vi "Accelerometer_status.vi"(6 "Number":i32, 10 "Acc_offset":dbl=0.0015, 11 "Accelerometer":sgl[](array[numeric])=array[5000 elements]) -> (2 "Accelerometer_status":string, 3 "Accelerometer":bool)   [LabVIEW 2015]
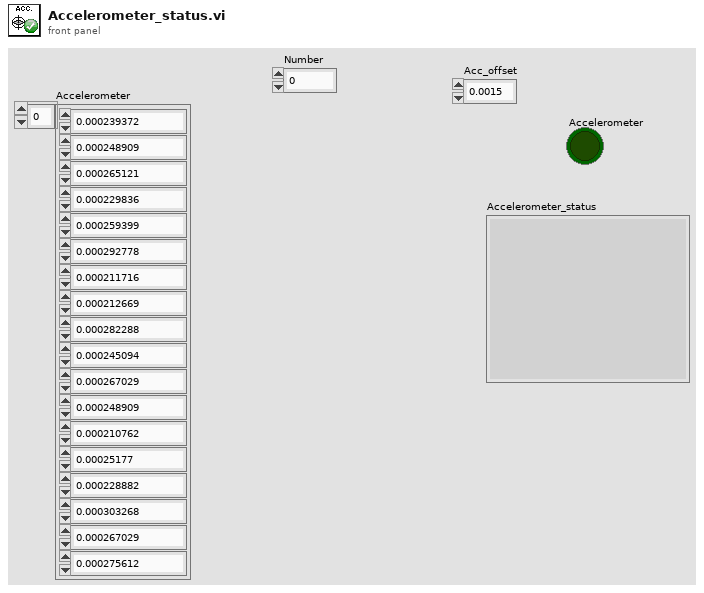
[diagram p1: front panel]
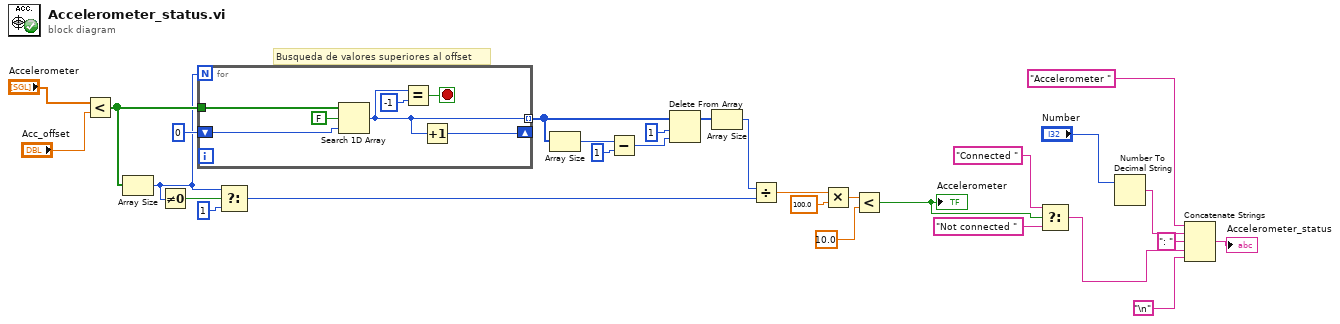
[diagram p0: block diagram]
diagram:
  # "Busqueda de valores superiores al offset"
  n1 = Less?(x="Accelerometer", y="Acc_offset") -> (x < y?=w29:bool[])
  n2 = Array Size(array=w29) -> (size(s)=w21:i32)
  n3 = Not Equal To 0?(x=w21) -> (x != 0?=w26:bool)
  n4 = for {
    N: w21 -> [_]
    tunnel: w29 -> [w36]
    tunnel: [w31] -> w15 mode=indexing
    shift-right: [w30] -> _
    shift-left: 0 ("index of element") -> [w32]
    stop <- w34 stop-if-true
    n5 = Search 1D Array(1D array=w36, element=FALSE, start index (0)=w32) -> (index of element=w31:i32)
    n6 = Equal?(x=w31, y=-1) -> (x = y?=w34:bool)
    n7 = Increment(x=w31) -> (x+1=w30:i32)
  }
  n8 = Select(t=w21, s=w26, f=1) -> (s? t:f=w27:i32)
  n9 = Array Size(array=w15) -> (size(s)=w19:i32)
  n10 = Subtract(x=w19, y=1 ("length")) -> (x-y=w17:i32)
  n11 = Delete From Array(array=w15, length=1, index=w17) -> (array with subset deleted=w14:i32[])  [unwired: 1 out]
  n12 = Array Size(array=w14) -> (size(s)=w22:i32)
  n13 = Divide(x=w22, y=w27) -> (x/y=w24:dbl)
  n14 = Multiply(x=w24, y=100.0) -> (x*y=w20:dbl)
  n15 = Less?(x=w20, y=10.0) -> (x < y?=w13:bool)
  "Accelerometer" <- w13
  n16 = Select(t="Connected " ("string"), s=w13, f="Not connected " ("string")) -> (s? t:f=w10:string)
  n17 = Number To Decimal String(number="Number") -> (decimal integer string=w3:string)  [unwired: 1 in]
  n18 = Concatenate Strings("Accelerometer " ("string"), w3, ": " ("string"), w10, "\n") -> (→"Accelerometer_status":string)
